vi "CG test stand DAQ main V2 LJ.vi"() -> ()   [LabVIEW 2020]
doc: "This example demonstrates how to read N channels of analog input from a LINX device."
uses:
  <vilib>/Analysis/Matrix/Numeric/Conversions/Array To Matrix - RA.vi
  <vilib>/Utility/file.llb/Write Delimited Spreadsheet (DBL).vi
  <vilib>/Analysis/Matrix/NI_Matrix.lvlib
panel:
  in  "?":T1(tab)
  in  "?":dbl
  out "A8_Scaled":dbl
  out "A7_Scaled":dbl
  out "A6_Scaled":dbl
  out "C1 8":dbl
  out "C2 8":dbl
  out "C3 8":dbl
  out "B 8":dbl
  out "C1 7":dbl
  out "C2 7":dbl
  out "C3 7":dbl
  out "B 7":dbl
  out "C1 6":dbl
  out "C2 6":dbl
  out "C3 6":dbl
  out "B 6":dbl
  out "C1 5":dbl
  out "C2 5":dbl
  out "C3 5":dbl
  out "B 5":dbl
  out "C1 4":dbl
  out "C2 4":dbl
  out "C3 4":dbl
  out "B 4":dbl
  out "C1 3":dbl
  out "C2 3":dbl
  out "C3 3":dbl
  out "B 3":dbl
  out "C1 2":dbl
  out "C2 2":dbl
  out "C3 2":dbl
  out "B 2":dbl
  out "C1 1":dbl
  out "C2 1":dbl
  out "C3 1":dbl
  out "B 1":dbl
  out "C1 0":dbl
  out "C2 0":dbl
  out "C3 0":dbl
  out "B 0":dbl
  out "A0_Scaled":dbl
  out "A1_Instrumentlabel":string
  out "A8_Voltage":dbl
  out "A8":dbl
  out "A7_Voltage":dbl
  out "A7":dbl
  out "A6_Voltage":dbl
  out "A6":dbl
  out "A5_Voltage":dbl
  out "A5":dbl
  out "A4_Voltage":dbl
  out "A4":dbl
  out "A3_Voltage":dbl
  out "A3":dbl
  out "A2_Voltage":dbl
  out "A2":dbl
  out "A1_Voltage":dbl
  out "A1":dbl
  out "A0_Voltage":dbl
  out "A0_Instrumentlabel":dbl
  out "A2_Instrumentlabel":string
  out "A3_Instrumentlabel":string
  out "A4_Instrumentlabel":string
  out "A5_Instrumentlabel":string
  out "A6_Instrumentlabel":string
  out "A7_Instrumentlabel":string
  out "A8_Instrumentlabel":string
  out "A0_Instrumentlabel 2":string
  out "A1_Scaled":dbl
  out "A2_Scaled":dbl
  out "A3_Scaled":dbl
  out "A4_Scaled":dbl
  out "A5_Scaled":dbl
  in  "DAC0":dbl format="%.4f"
  in  "FIO6":bool
  in  "FIO7":bool
  out "Error Message":string
  out "LABJACK U3 Error":errorcluster
  out "Value 2":dbl
  out "Resistance":dbl
  out "Temp":dbl
  in  "C":dbl
  in  "P0 Port":dbl
  in  "P0 Label":string
  out "?":dbl(graph)
  in  "P0 A":dbl
  in  "P0 B":dbl
  out "?":dbl(graph)
  in  "P0 Label 2":string
  in  "P0 Port 2":dbl
  in  "P0 A 2":dbl
  in  "P0 B 2":dbl
  out "?":dbl(graph)
  in  "P0 Label 3":string
  in  "P0 Port 3":dbl
  in  "A":dbl
  in  "B":dbl
  out "?":dbl(graph)
  in  "P0 Label 4":string
  in  "P0 Port 4":dbl
  in  "P0 A 4":dbl
  in  "P0 B 4":dbl
  out "Value":dbl
  out "Filtered Voltage":dbl(graph)
  out "Unfiltered Voltage":dbl
  out "Filtered Voltage":dbl
  in  "Filtered Port":u32
  out "Venturi Thrust":dbl(knob) scale=0.0..1000.0
  out "Data Rate (Hz)":dbl
  out "?":dbl
  out "?":dbl
  out "?":dbl
  out "Thrust":dbl(graph)
  out "Orifice Pressure":dbl(knob) scale=0.0..160.0
  out "Reg Pressure":dbl(knob) scale=0.0..10.0
  out "Orifice inlet pressure":dbl(graph)
  out "Tank Pressure":dbl(knob) scale=0.0..3000.0
  in  "Interval (ms)":u32
  in  "?":bool
  in  "Stop Button":bool
  out "WRITING TO FILE":bool
  out "error out":errorcluster
  out "Full filepath":string
  in  "Path":path
  in  "File extension":string
  in  "Filename":string
  out "Time Stamp":timestamp
  in  "Calibration Value":dbl
  # "Analog Inputs"
  # "Tare value"
  # "Analog Port"
  # "Voltage In"
  # "X3"
  # "X2"
  # "X1"
  # "B"
  # "Instrument name"
  # "Scaled Value"
  # "X+"
  # "X+"
  # "X+"
  # "File I/O"
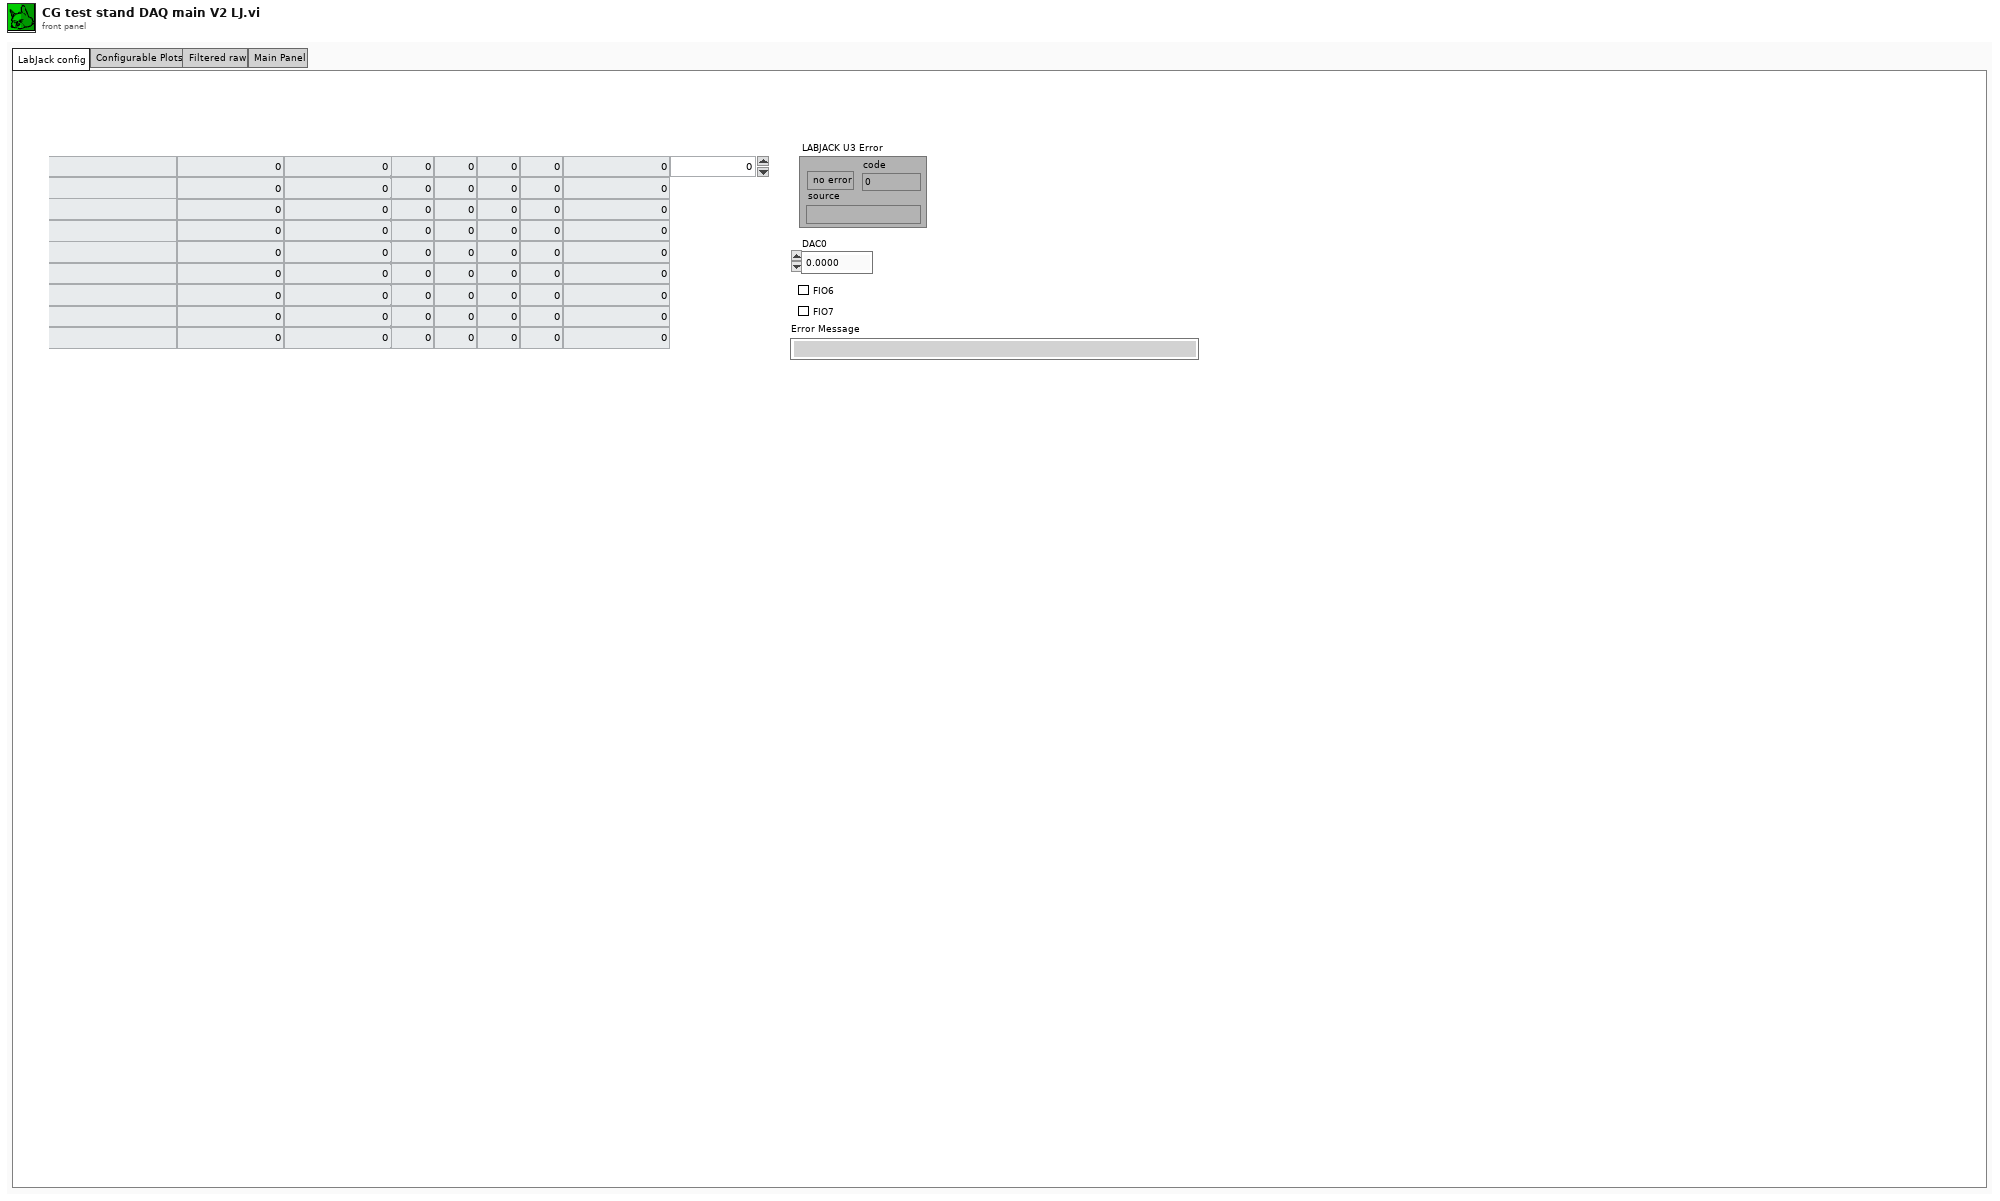
[diagram p1: front panel]
types:
  T1 = enum32{"LabJack config", "Configurable Plots", "Filtered raw", "Main Panel"}
  T2 = typedef "NI_Matrix.lvlib/RealMatrix.ctl" = dbl[][]
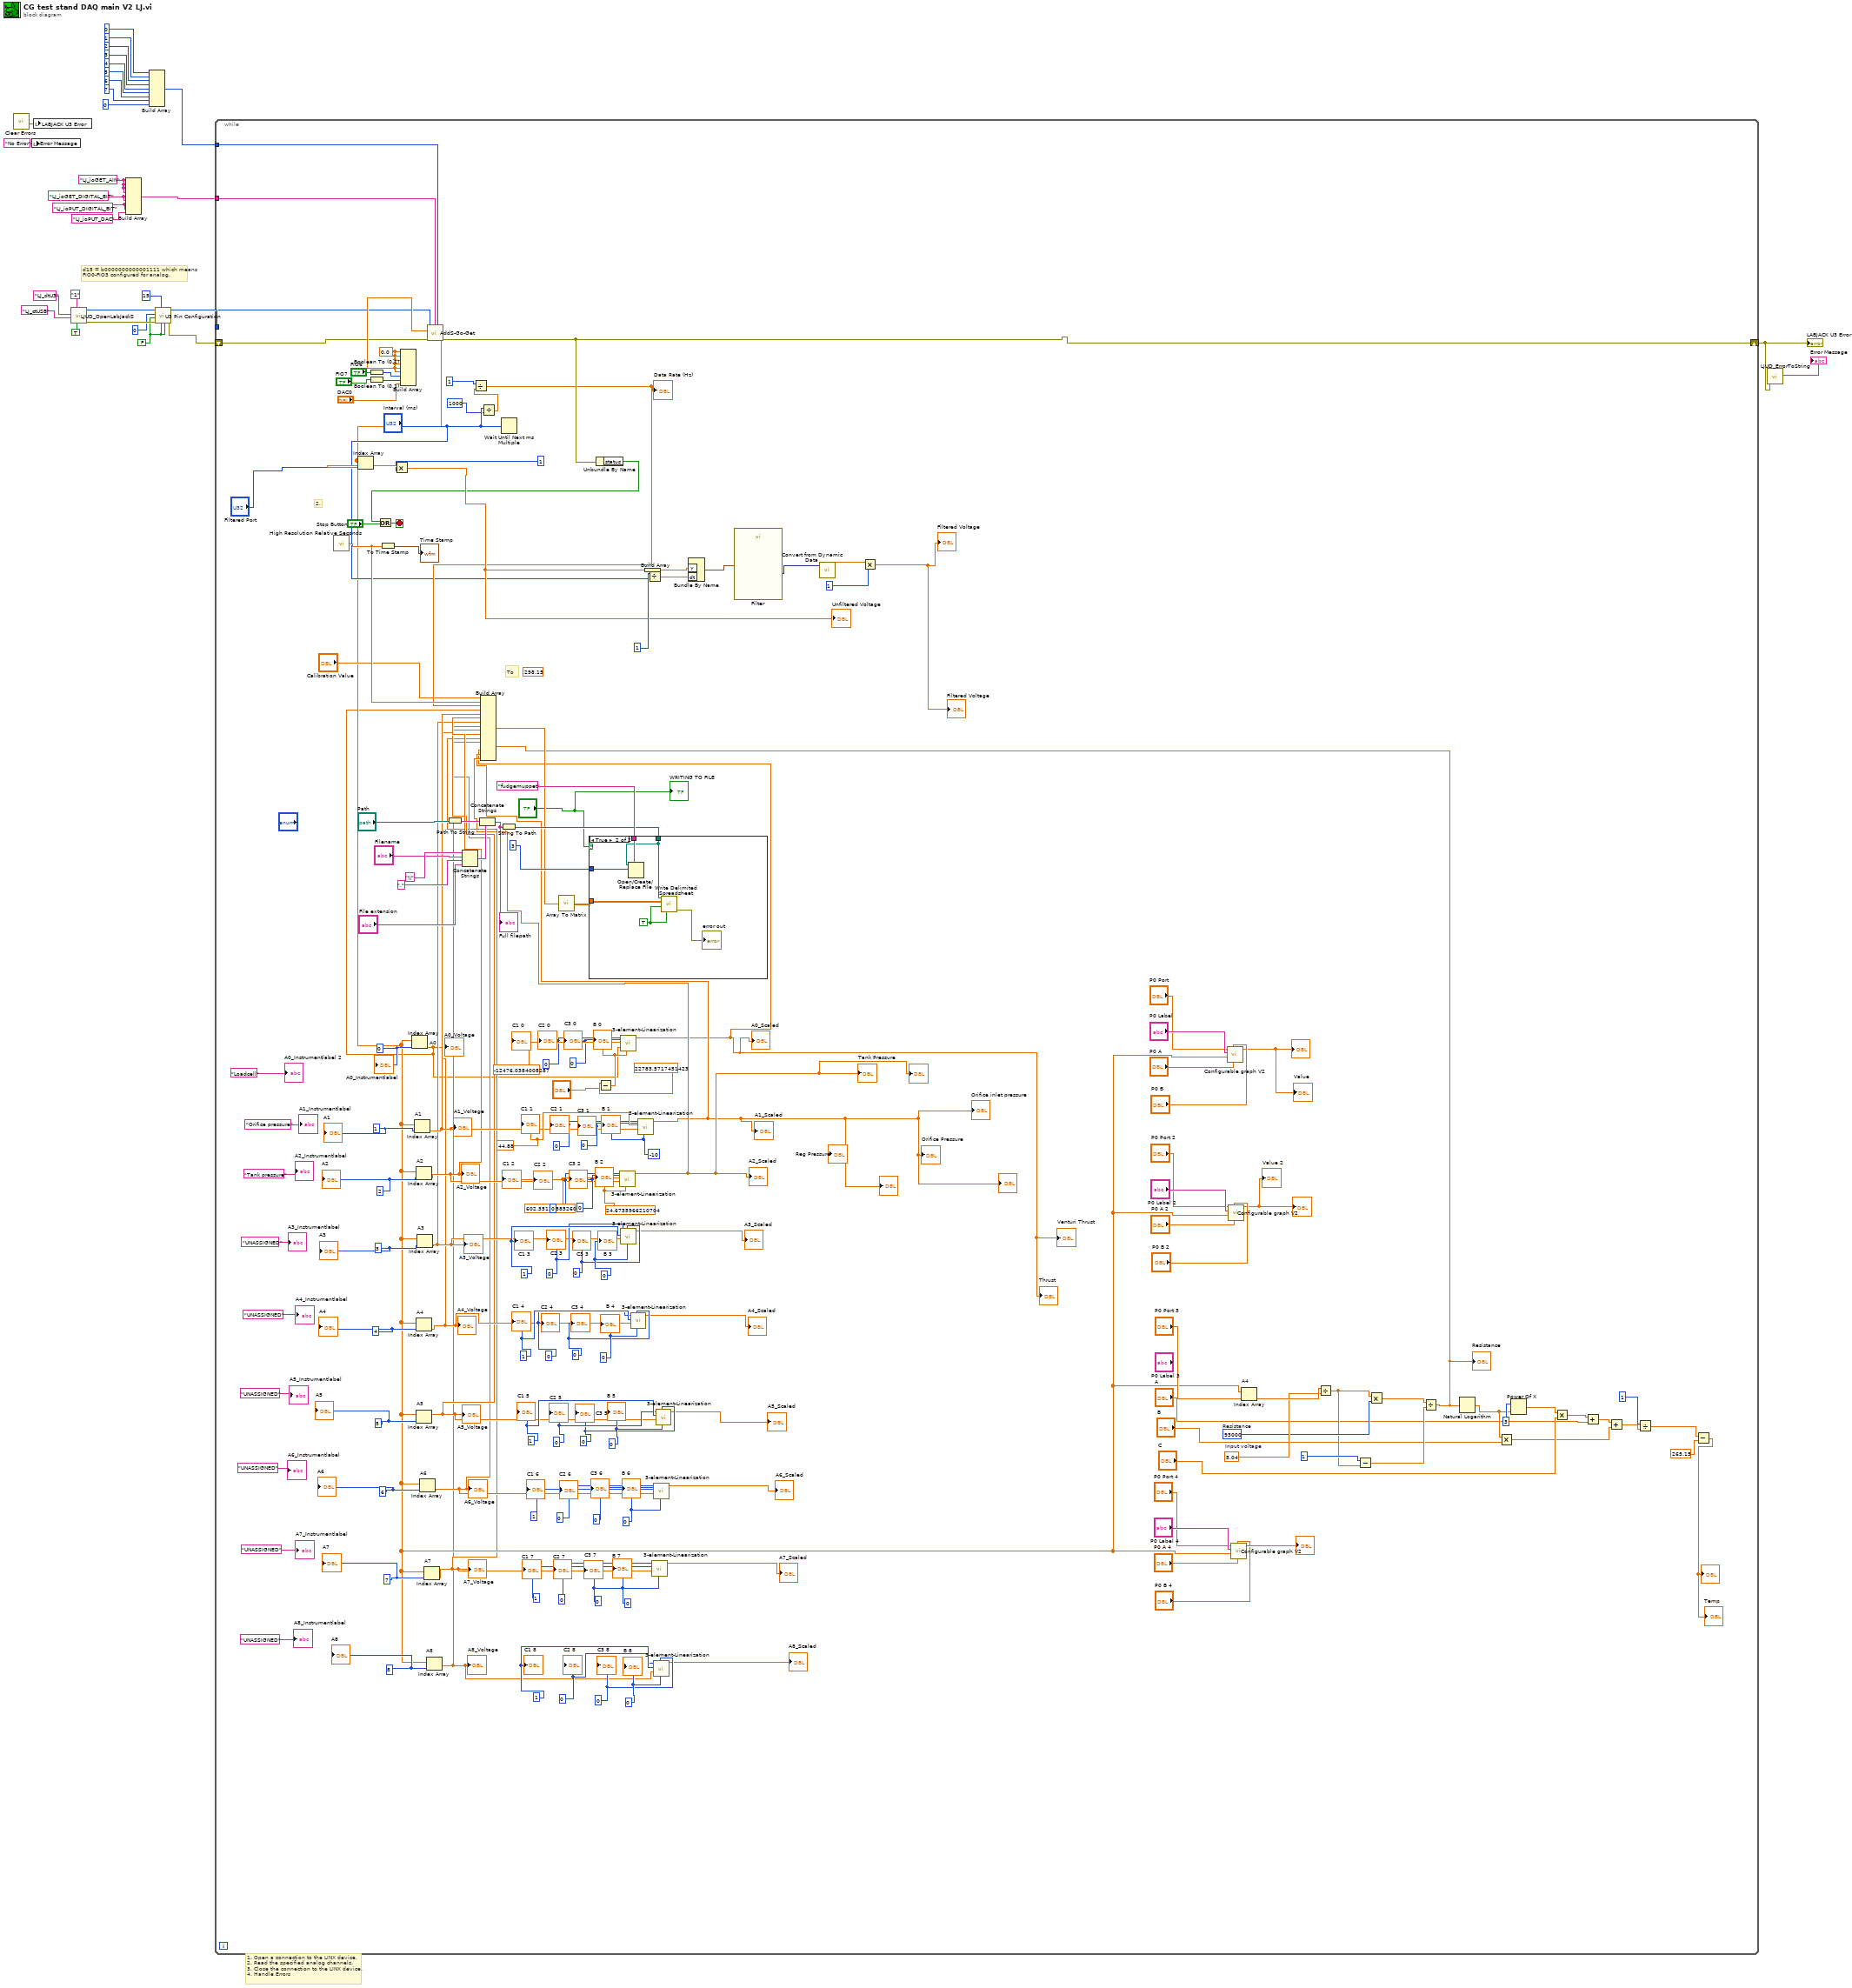
[diagram p0: block diagram]
diagram:
  w17 = "LJ_ioPUT_DIGITAL_BIT" ("IOType")
  w19 = "LJ_ioGET_AIN" ("IOType")
  w18 = "LJ_ioGET_DIGITAL_BIT" ("IOType")
  w22 = FALSE ("Enable DAC1")
  # "d15 = b0000000000001111 which means\nFIO0-FIO3 configured for analog."
  # "1. Open a connection to the LINX device.\n2. Read the specified analog channels.\n3. Close the connection to the LINX device.\n4. Handle Errors"
  n1 = call <vilib>:"Clear Errors.vi"() -> ("error out"=w5:errorcluster)  [unwired: 6 in, 1 out]
  n2 = local write "Error Message"("No Error" ("Error Message")) -> ()
  n3 = local write "LABJACK U3 Error"(w5) -> ()
  n4 = call <vilib>:"LJUD_OpenLabJackS.vi"("FirstFound"=TRUE, "Address"="1", "ConnectionType"="LJ_ctUSB", "DeviceType"="LJ_dtU3") -> ("error out"=w26:errorcluster, "Handle"=w25:i32)  [unwired: 5 in, 1 out]
  n5 = Build Array(w19, w19, w19, w19, w18, w18, w17, w17, "LJ_ioPUT_DAC" ("IOType")) -> (w2:string[])
  n6 = Build Array(0, 1, 2, 3, 4, 5, 6, 7, 0) -> (w1:i32[])
  n7 = call <vilib>:"U3 Pin Configuration.vi"("Enable Counter1"=w22, "Enable Counter0"=w22, "FIO/EIO Analog Enable"=15, "error in"=w26, "Enable DAC1"=w22, "Number of Timers Enabled"=u8 0, "Handle In"=w25) -> ("error out"=w20:errorcluster, "Handle Out"=w21:i32)  [unwired: 3 in]
  n8 = while {
    tunnel: w21 -> [w100]
    shift-right: [w98] -> w3
    shift-left: w20 -> [w99]
    tunnel: w2 -> [w96]
    tunnel: w1 -> [w95]
    stop <- w192 stop-if-true
    w69 = 5.04  # Input voltage
    w68 = 93000  # Resistance
    w106 = 0.0 ("Input Element")
    w119 = 0
    w116 = 0
    w117 = 0
    w118 = 1
    w124 = 0
    w121 = 0
    w122 = 0
    w123 = 1
    w129 = 0
    w126 = 0
    w127 = 0
    w128 = 1
    w114 = 0
    w111 = 0
    w112 = 0
    w113 = 1
    w133 = 0
    w130 = 0
    w131 = 0
    w132 = 1
    w137 = 0
    w134 = 0
    w135 = 0
    w136 = 1
    w141 = 24.6735966210704
    w138 = 0
    w139 = 0
    w140 = 602.351358852601
    w38 = -10
    w142 = 0
    w143 = 0
    w144 = 44.88
    w145 = 0
    w146 = 0
    w147 = -12476.0384008287
    w157 = 8
    w158 = 7
    w159 = 6
    w160 = 5
    w161 = 4
    w163 = 3
    w162 = 2
    w164 = 1
    w165 = 0
    (unwired) 298.15
    # "To"
    # "2."
    n9 = call <vilib>:"High Resolution Relative Seconds.vi"() -> ("relative seconds"=w189:dbl)
    n10 = Boolean To (0,1)(Boolean="FIO6") -> (0, 1=w105:i16)
    n11 = Boolean To (0,1)(Boolean="FIO7") -> (0, 1=w104:i16)
    n12 = To Time Stamp(1:w189) -> (0:→"Time Stamp":timestamp)
    n13 = Build Array(w106, w106, w106, w106, w106, w106, w105, w104, "DAC0") -> (w103:dbl[])
    n14 = call <vilib>:"AddS-Go-Get.vi"("Channels"=w95, "IOTypes"=w96, "error in"=w99, "Values Write"=w103, "Handle In"=w100) -> ("error out"=w98:errorcluster, "Values Read"=w71:dbl[])  [unwired: 4 in, 1 out]
    n15 = Index Array(array=w71, index="Filtered Port") -> (element=w184:dbl)
    n16 = Multiply(x=w184, y=1) -> (x*y=w179:dbl)
    "Unfiltered Voltage" <- w179
    n17 = Index Array "A0"(array=w71, index=w165) -> (element=w35:dbl)
    "A0_Voltage" <- w35
    n18 = Index Array "A1"(array=w71, index=w164) -> (element=w51:dbl)
    "A1_Voltage" <- w51
    n19 = Index Array "A2"(array=w71, index=w162) -> (element=w50:dbl)
    "A2_Voltage" <- w50
    n20 = Index Array "A4"(array=w71, index=w161) -> (element=w48:dbl)
    "A4_Voltage" <- w48
    n21 = Index Array "A5"(array=w71, index=w160) -> (element=w47:dbl)
    "A5_Voltage" <- w47
    n22 = Index Array "A3"(array=w71, index=w163) -> (element=w49:dbl)
    "A3_Voltage" <- w49
    n23 = Index Array "A6"(array=w71, index=w159) -> (element=w46:dbl)
    "A6_Voltage" <- w46
    n24 = Index Array "A7"(array=w71, index=w158) -> (element=w45:dbl)
    "A7_Voltage" <- w45
    n25 = Index Array "A8"(array=w71, index=w157) -> (element=w44:dbl)
    "A8_Voltage" <- w44
    n26 = Path To String(path="Path") -> (string=w173:string)
    n27 = Concatenate Strings("\\", "Filename", ".", "File extension") -> (w166:string)
    n28 = Concatenate Strings(w173, w166) -> (w174:string)
    "Full filepath" <- w174
    n29 = Divide(x="Interval (ms)", y=1000) -> (x/y=w90:dbl)
    n30 = Divide(x=1, y=w90) -> (x/y=w93:dbl)
    "Data Rate (Hz)" <- w93
    n31 = String To Path(string=w174) -> (path=w175:path)
    n32 = Wait Until Next ms Multiple(millisecond multiple="Interval (ms)") -> ()  [unwired: 1 out]
    n33 = Unbundle By Name(w98) -> ("status"=w107:bool)
    n34 = Or(x=w107, y="Stop Button") -> (x .or. y?=w192:bool)
    n35 = Subtract(x=22783.5717451423, y="?") -> (x-y=w88:dbl)
    "B 0" <- w88
    n36 = call "3-element-Linearization.vi"("B"=w141, "C3"=w138, "Voltage in"=w50, "C1"=w140, "C2"=w139) -> ("Scaled value"=w34:dbl)  [unwired: 6 in]
    "A2_Scaled" <- w34
    "Tank Pressure" <- w34
    "?" <- w34
    n37 = call "3-element-Linearization.vi"("B"=w88, "C3"=w145, "Voltage in"=w35, "C1"=w147, "C2"=w146) -> ("Scaled value"=w32:dbl)  [unwired: 6 in]
    "A0_Scaled" <- w32
    "Thrust" <- w32
    "Venturi Thrust" <- w32
    n38 = call "3-element-Linearization.vi"("B"=w137, "C3"=w134, "Voltage in"=w49, "C1"=w136, "C2"=w135) -> ("Scaled value"=→"A3_Scaled":dbl)  [unwired: 6 in]
    n39 = call "3-element-Linearization.vi"("B"=w133, "C3"=w130, "Voltage in"=w48, "C1"=w132, "C2"=w131) -> ("Scaled value"=→"A4_Scaled":dbl)  [unwired: 6 in]
    n40 = call "3-element-Linearization.vi"("B"=w38, "C3"=w142, "Voltage in"=w51, "C1"=w144, "C2"=w143) -> ("Scaled value"=w33:dbl)  [unwired: 6 in]
    "A1_Scaled" <- w33
    "Orifice inlet pressure" <- w33
    "Reg Pressure" <- w33
    "Orifice Pressure" <- w33
    "?" <- w33
    "?" <- w33
    n41 = Build Array(w179) -> (w186:dbl[])
    n42 = Divide(x=1, y="Interval (ms)") -> (x/y=w188:dbl)
    n43 = call "3-element-Linearization.vi"("B"=w124, "C3"=w121, "Voltage in"=w45, "C1"=w123, "C2"=w122) -> ("Scaled value"=→"A7_Scaled":dbl)  [unwired: 6 in]
    n44 = call "3-element-Linearization.vi"("B"=w129, "C3"=w126, "Voltage in"=w46, "C1"=w128, "C2"=w127) -> ("Scaled value"=→"A6_Scaled":dbl)  [unwired: 6 in]
    n45 = call "3-element-Linearization.vi"("B"=w119, "C3"=w116, "Voltage in"=w44, "C1"=w118, "C2"=w117) -> ("Scaled value"=→"A8_Scaled":dbl)  [unwired: 6 in]
    n46 = call "3-element-Linearization.vi"("B"=w114, "C3"=w111, "Voltage in"=w47, "C1"=w113, "C2"=w112) -> ("Scaled value"=→"A5_Scaled":dbl)  [unwired: 6 in]
    n47 = Bundle By Name("Y"=w186, "dt"=w188) -> (w185:waveform(dbl))  [unwired: 1 in]
    n48 = call "Filter"("Signal"=w185) -> ("Filtered Signal"=w182:dynamicdata)  [unwired: 9 in, 1 out]
    n49 = call "Convert from Dynamic Data"("Dynamic Data Type"=w182) -> ("Scalar"=w181:dbl)  [unwired: 3 in]
    n50 = Multiply(x=w181, y=1) -> (x*y=→"Filtered Voltage" →"Filtered Voltage":dbl)
    n51 = call "Configurable graph V2.vi"("A"="P0 A", "B"="P0 B", "Input Voltages"=w71, "Instrument Label"="P0 Label", "Port #"="P0 Port") -> ("Scaled output"=→"?" →"Value":dbl)  [unwired: 6 in]
    n52 = call "Configurable graph V2.vi"("A"="P0 A 2", "B"="P0 B 2", "Input Voltages"=w71, "Instrument Label"="P0 Label 2", "Port #"="P0 Port 2") -> ("Scaled output"=→"?" →"Value 2":dbl)  [unwired: 6 in]
    n53 = call "Configurable graph V2.vi"("A"="P0 A 4", "B"="P0 B 4", "Input Voltages"=w71, "Instrument Label"="P0 Label 4", "Port #"="P0 Port 4") -> ("Scaled output"=→"?":dbl)  [unwired: 6 in]
    n54 = Index Array "A4"(array=w71, index="P0 Port 3") -> (element=w70:dbl)
    n55 = Divide(x=w70, y=w69) -> (x/y=w65:dbl)
    n56 = Subtract(x=1, y=w65) -> (x-y=w64:dbl)
    n57 = Multiply(x=w65, y=w68) -> (x*y=w67:dbl)
    n58 = Divide(x=w67, y=w64) -> (x/y=w40:dbl)
    "Resistance" <- w40
    n59 = Build Array("Calibration Value", w189, w93, w35, w51, w50, w49, w48, w47, w46, w45, w44, w40, w32, w33, w34) -> (w171:dbl[])
    n60 = call-poly <vilib>:"Array To Matrix.vi"("Real 1D Array"=w171) -> ("Real Matrix (Column Vector)"=w178:T2)
    n61 = case shown="True" "?" {
      tunnel: w175 -> [_ w196]
      tunnel: w178 -> [_ w193]
      tunnel: "fudgemuppet" -> [_ w198]
      tunnel: 3 -> [_ w197]
      frame False {
      }
      frame True {
        w194 = TRUE
        n62 = Open/Create/Replace File(file path (use dialog)=w196, prompt=w198, operation (0:open)=w197) -> ()  [unwired: 3 in, 3 out]
        n63 = call-poly <vilib>:"Write Delimited Spreadsheet.vi"("file path (dialog if empty)"=w196, "2D data"=w193, "append to file? (new file:F)"=w194, "transpose? (no:F)"=w194) -> ("error out"=→"error out":errorcluster)  [unwired: 10 in, 1 out]
      }
    }
    n64 = Natural Logarithm(1:w40) -> (0:w60:dbl)
    n65 = Multiply(x=w60, y="B") -> (x*y=w55:dbl)
    n66 = Power Of X(1:w60, 2:3) -> (0:w62:dbl)
    n67 = Multiply(x=w62, y="C") -> (x*y=w58:dbl)
    n68 = Add(x=w58, y="A") -> (x+y=w56:dbl)
    n69 = Add(x=w56, y=w55) -> (x+y=w54:dbl)
    n70 = Divide(x=1, y=w54) -> (x/y=w43:dbl)
    n71 = Subtract(x=w43, y=265.15) -> (x-y=→"?" →"Temp":dbl)
    "WRITING TO FILE" <- "?"
    "A0_Instrumentlabel" <- w165
    "A1" <- w164
    "A2" <- w162
    "A3" <- w163
    "A4" <- w161
    "A5" <- w160
    "A6" <- w159
    "A7" <- w158
    "A8" <- w157
    "A1_Instrumentlabel" <- "Orifice pressure"
    "A2_Instrumentlabel" <- "Tank pressure"
    "A3_Instrumentlabel" <- "UNASSIGNED"
    "A4_Instrumentlabel" <- "UNASSIGNED"
    "A5_Instrumentlabel" <- "UNASSIGNED"
    "A6_Instrumentlabel" <- "UNASSIGNED"
    "A7_Instrumentlabel" <- "UNASSIGNED"
    "A8_Instrumentlabel" <- "UNASSIGNED"
    "A0_Instrumentlabel 2" <- "Loadcell"
    "C3 0" <- w145
    "C2 0" <- w146
    "C1 0" <- w147
    "B 1" <- w38
    "C3 1" <- w142
    "C2 1" <- w143
    "C1 1" <- w144
    "B 2" <- w141
    "C3 2" <- w138
    "C2 2" <- w139
    "C1 2" <- w140
    "B 3" <- w137
    "C3 3" <- w134
    "C2 3" <- w135
    "C1 3" <- w136
    "B 4" <- w133
    "C3 4" <- w130
    "C2 4" <- w131
    "C1 4" <- w132
    "B 5" <- w114
    "C3 5" <- w111
    "C2 5" <- w112
    "C1 5" <- w113
    "B 6" <- w129
    "C3 6" <- w126
    "C2 6" <- w127
    "C1 6" <- w128
    "B 7" <- w124
    "C3 7" <- w121
    "C2 7" <- w122
    "C1 7" <- w123
    "B 8" <- w119
    "C3 8" <- w116
    "C2 8" <- w117
    "C1 8" <- w118
  }
  "LABJACK U3 Error" <- w3
  n72 = call <vilib>:"LJUD_ErrorToString.vi"("error in"=w3) -> ("String"=→"Error Message":string)  [unwired: 10 in]
